vi "Entry.vi"(8 "error in (no error)":errorcluster, 11 "New State":refnum<class "Numeric.lvclass">) -> (0 "error out":errorcluster, 3 "State out":refnum<class "Numeric.lvclass">)   [LabVIEW 2020, in "Keypad.lvlib" / "Numeric.lvclass"]
doc: "This is an abstract method. Override this method to define the behavior when you enter the state."
uses:
  Numeric.lvclass
  Keypad/Keypad.lvclass
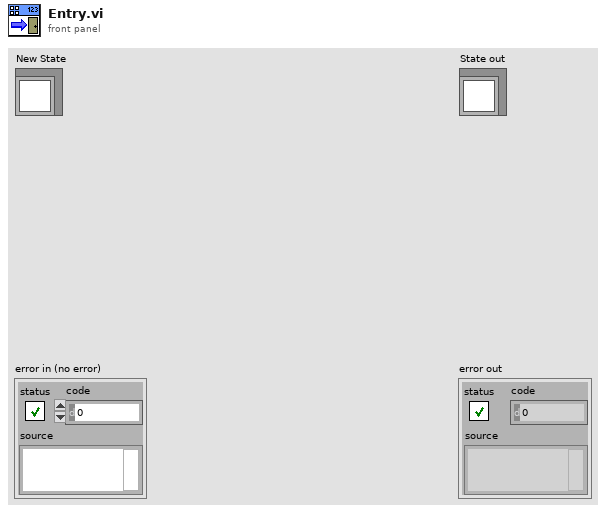
[diagram p1: front panel]
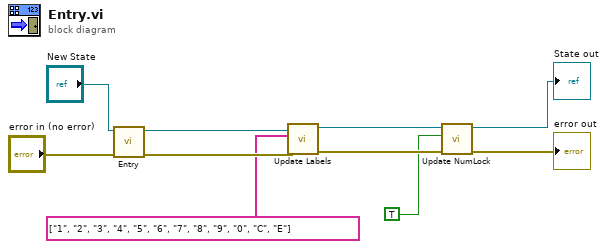
[diagram p0: block diagram]
diagram:
  n1 = call-parent "Entry.vi"("error in (no error)"="error in (no error)", "New State"="New State") -> ("error out"=w7:errorcluster, "State out"=w8:refnum<class "Numeric.lvclass">)  [unwired: 8 in]
  n2 = call "Update Labels.vi"("error in (no error)"=w7, "Labels"=string[] ["1", "2", "3", "4", "5", "6", "7", "8", "9", "0", "C", "E"], "Keypad in"=w8) -> ("error out"=w5:errorcluster, "Keypad out"=w6:refnum<class "Numeric.lvclass">)  [unwired: 7 in]
  n3 = call "Update NumLock.vi"("error in (no error)"=w5, "NuLockS State"=TRUE, "Keypad in"=w6) -> ("error out"=→"error out":errorcluster, "Keypad out"=→"State out":refnum<class "Numeric.lvclass">)  [unwired: 7 in]
